vi "_FPGA Check Door.vi"(4 "error in":errorcluster, 5 "DisableCheck (F)":bool, 6 "CheckNow (F)":bool) -> (0 "error out":errorcluster, 2 "DoorOK":bool)   [LabVIEW 2015]
uses:
  Type/_RW Status.ctl
  Type/_LED States.ctl
  Type/_LCD Line2 Msg.ctl
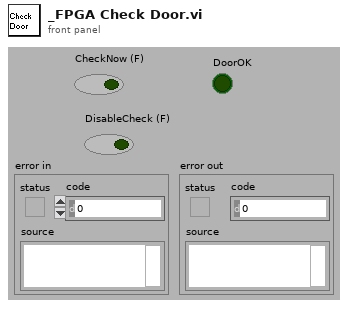
[diagram p1: front panel]
types:
  T1 = typedef "_LED States.ctl" = enum8{"Idle", "Solid B", "Solid R", "Solid P", "Off B", "Off R", "Off P", "Off BRP", "Off RP", "Flash R&P", "Flash P"}
  T2 = typedef "_RW Status.ctl" = enum8{"Done", "Do Read", "Do Write", "Set Latch1", "Set Latch2", "Set Latch3", "Set Latch4", "RP ON", "EL ON", "Serial Send", "Set LC Out", "Get LC In", "Read VAC", "Table Test", "Get Interlock", "Do Read2", "Do Write2"}
  T3 = typedef "_LCD Line2 Msg.ctl" = u16
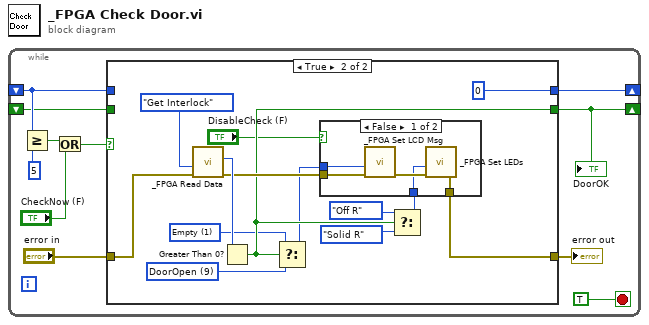
[diagram p0: block diagram]
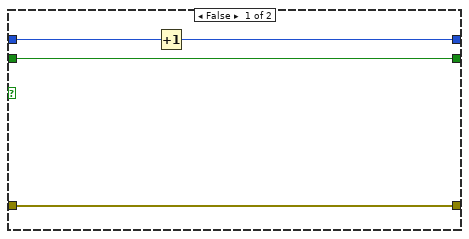
[diagram p2: hidden frame]
diagram:
  n1 = while {
    shift-right: [w10] -> _
    shift-left: _ -> [w5]
    shift-right: [w1] -> _
    shift-left: _ -> [w2]
    stop <- TRUE stop-if-true
    n2 = Greater Or Equal?(x=w5, y=5) -> (x >= y?=w8:bool)
    n3 = Or(x=w8, y="CheckNow (F)") -> (x .or. y?=w6:bool)
    n4 = case shown="True" w6 {
      tunnel: [w14 0] -> w10
      tunnel: w5 -> [w15 _]
      tunnel: [w13 w20] -> w3
      tunnel: "error in" -> [w13 w26]
      tunnel: [w12 w24] -> w1
      tunnel: w2 -> [w12 _]
      frame False {
        n5 = Increment(x=w15) -> (x+1=w14:i32)
      }
      frame True {
        w19 = T3 9 items=["Same", "Empty", "VacFail", "Cancel", "CheckGas", "EleFail", "Probe1Fail", "Probe2Fail", "HeaterFail", "DoorOpen", "CheckComm", "PressStart"] ("Line2Msg (same)")
        w18 = T3 1 items=["Same", "Empty", "VacFail", "Cancel", "CheckGas", "EleFail", "Probe1Fail", "Probe2Fail", "HeaterFail", "DoorOpen", "CheckComm", "PressStart"] ("Line2Msg (same)")
        n6 = call "_FPGA Read Data.vi"("error in"=w26, "Read Mode (Do Read)"=_RW_Status."Get Interlock" ("R/W Status")) -> ("error out"=w25:errorcluster, "Data"=w28:u32)  [unwired: 3 in, 1 out]
        n7 = Greater Than 0?(x=w28) -> (x > 0?=w24:bool)
        n8 = Select(t=w18, s=w24, f=w19) -> (s? t:f=w17:T3)
        n9 = Select(t=_LED_States."Off R" ("LED Command"), s=w24, f=_LED_States."Solid R" ("LED Command")) -> (s? t:f=w21:T1)
        n10 = case shown="False" "DisableCheck (F)" {
          tunnel: w25 -> [w34 w35]
          tunnel: w21 -> [w32 _]
          tunnel: [w31 w35] -> w20
          tunnel: w17 -> [w30 _]
          frame False {
            n11 = call "_FPGA Set LCD Msg.vi"("error in"=w34, "Line2Msg (same)"=w30) -> ("error out"=w33:errorcluster)  [unwired: 5 in, 2 out]
            n12 = call "_FPGA Set LEDs.vi"("error in (no error)"=w33, "LED Command"=w32) -> ("error out"=w31:errorcluster)  [unwired: 2 in, 3 out]
          }
          frame True {
          }
        }
      }
    }
    "error out" <- w3
    "DoorOK" <- w1
  }
